vi "步响应起始点_V2.vi"(3 "（要求）连续大于0的次数":dbl=100.0, 4 "rise_step":dbl=10.0, 5 "行程 in":dbl[](array[numeric])) -> (1 "X_value":dbl, 2 "行程 out":dbl[](array[numeric]))   [LabVIEW 2013]
panel:
  out "连续大于0的次数":dbl=10.0
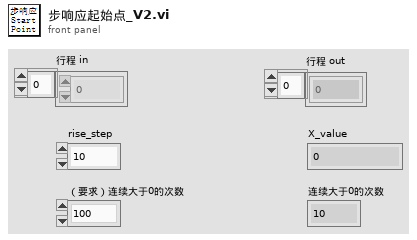
[diagram p1: front panel]
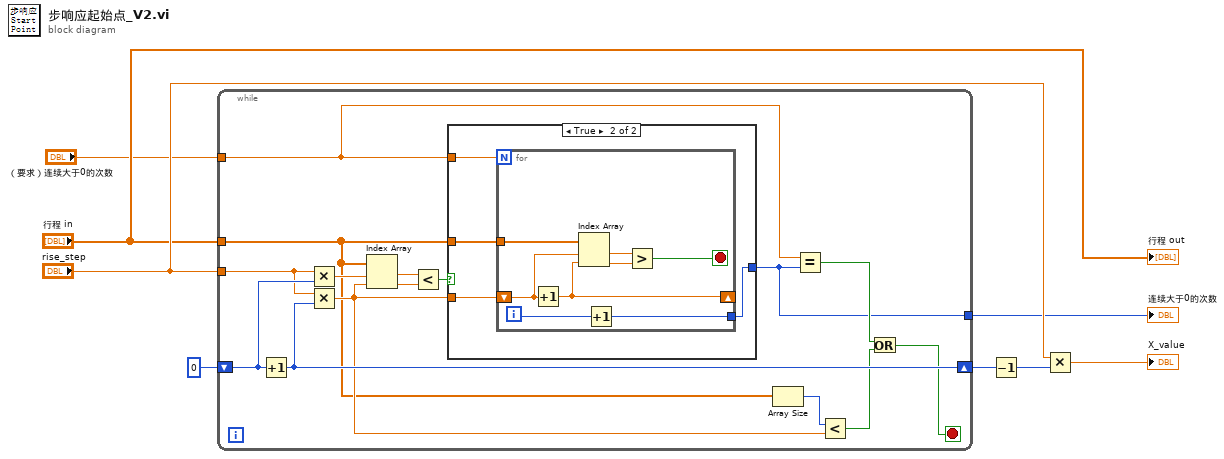
[diagram p0: block diagram]
diagram:
  n1 = while {
    tunnel: "rise_step" -> [w17]
    tunnel: "行程 in" -> [w12]
    shift-right: [w21] -> w4
    shift-left: 0 -> [w22]
    tunnel: "（要求）连续大于0的次数" -> [w11]
    tunnel: [w9] -> w1
    stop <- w19 stop-if-true
    n2 = Increment(x=w22) -> (x+1=w21:i32)
    n3 = Multiply(x=w17, y=w22) -> (x*y=w23:dbl)
    n4 = Multiply(x=w17, y=w21) -> (x*y=w13:dbl)
    n5 = Index Array(array=w12, index #1=w23, index #2=w13) -> (element #1=w15:dbl, element #2=w16:dbl)
    n6 = Less?(x=w15, y=w16) -> (x < y?=w14:bool)
    n7 = case shown="True" w14 {
      tunnel: w11 -> [_ w27]
      tunnel: w13 -> [_ w26]
      tunnel: w12 -> [_ w25]
      tunnel: [_ w24] -> w9
      frame False {
      }
      frame True {
        n8 = for {
          N: w27 -> [_]
          shift-right: [w35] -> _
          shift-left: w26 -> [w34]
          tunnel: w25 -> [w31]
          tunnel: [w28] -> w24
          i -> [w29]
          stop <- w30 stop-if-true
          n9 = Increment(x=w34) -> (x+1=w35:dbl)
          n10 = Index Array(array=w31, index #1=w34, index #2=w35) -> (element #1=w33:dbl, element #2=w32:dbl)
          n11 = Increment(x=w29) -> (x+1=w28:i32)
          n12 = Greater?(x=w33, y=w32) -> (0:w30:bool)
        }
      }
    }
    n13 = Array Size(array=w12) -> (size(s)=w20:i32)
    n14 = Equal?(x=w11, y=w9) -> (x = y?=w10:bool)
    n15 = Less?(x=w20, y=w13) -> (x < y?=w18:bool)
    n16 = Or(x=w10, y=w18) -> (x .or. y?=w19:bool)
  }
  "连续大于0的次数" <- w1
  n17 = Decrement(x=w4) -> (x-1=w3:i32)
  n18 = Multiply(x="rise_step", y=w3) -> (x*y=→"X_value":dbl)
  "行程 out" <- "行程 in"
